vi "Read Asynchronous Measurement (Resistance).vi"(6 "Wait Time (10 S)":i32=10, 8 "error in (no error)":errorcluster, 9 "Resistance Buffer (smua.nvbuffer1)":string="smua.nvbuffer1", 10 "Source Measure Unit Channel (0: Channel A)":i32(ring) items=["Channel A", "Channel B"], 11 "VISA resource name":refnum<visa-resource-name>) -> (0 "error out":errorcluster, 2 "Resistance Buffer Data (Ohm)":dbl[](array[numeric]), 3 "VISA resource name out":refnum<visa-resource-name>)   [LabVIEW 2019, in "Keithley 2600 Series.lvlib"]
doc: "Returns the asynchronous resistance measurements."
uses:
  Keithley 2600 Series.lvlib
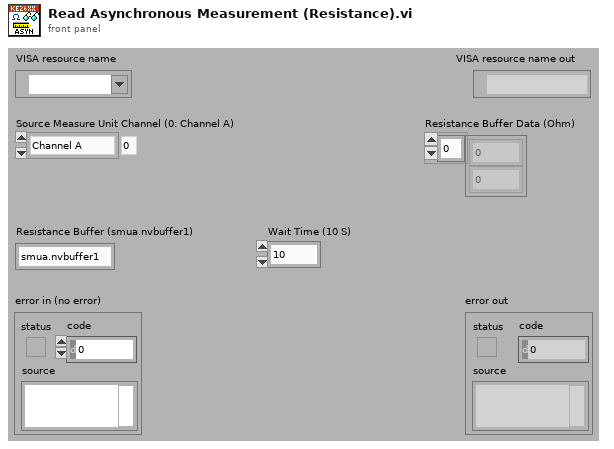
[diagram p1: front panel]
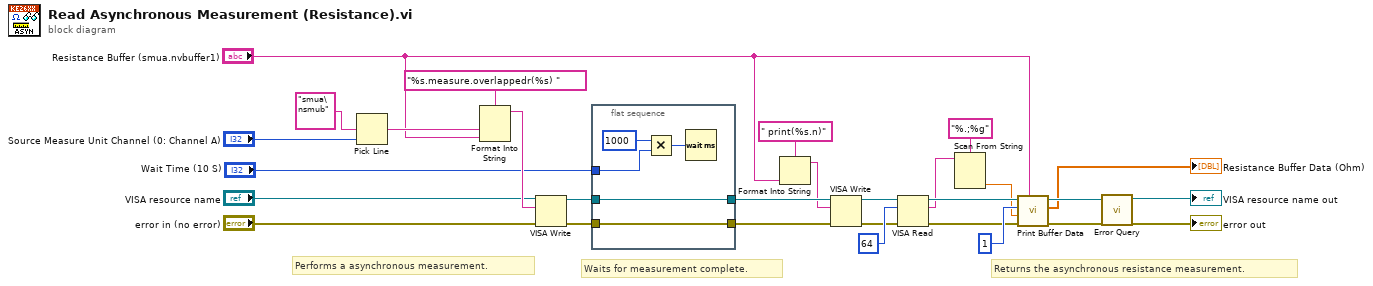
[diagram p0: block diagram]
diagram:
  # "Performs a asynchronous measurement."
  # "Waits for measurement complete."
  # "Returns the asynchronous resistance measurement."
  n1 = Pick Line(multi-line string="smua\nsmub", line index="Source Measure Unit Channel (0: Channel A)") -> (output string=w20:string)  [unwired: 1 in]
  n2 = Format Into String(format string="%s.measure.overlappedr(%s) ", w20, "Resistance Buffer (smua.nvbuffer1)") -> (resulting string=w26:string)  [unwired: 2 in, 1 out]
  n3 = VISA Write(VISA resource name="VISA resource name", write buffer=w26, error in (no error)="error in (no error)") -> (VISA resource name out=w10:refnum<visa-resource-name>, error out=w9:errorcluster)  [unwired: 1 out]
  n4 = flat-sequence {
    tunnel: w10 -> [w34]
    tunnel: w9 -> [w33]
    tunnel: [w34] -> w8
    tunnel: [w33] -> w7
    tunnel: "Wait Time (10 S)" -> [w32]
    frame #0 {
      n5 = Multiply(x=u32 1000, y=w32) -> (x*y=w30:u32)
      n6 = Wait (ms)(milliseconds to wait=w30) -> ()  [unwired: 1 out]
    }
  }
  n7 = Format Into String(format string=" print(%s.n)", "Resistance Buffer (smua.nvbuffer1)") -> (resulting string=w2:string)  [unwired: 2 in, 1 out]
  n8 = VISA Write(VISA resource name=w8, write buffer=w2, error in (no error)=w7) -> (VISA resource name out=w6:refnum<visa-resource-name>, error out=w5:errorcluster)  [unwired: 1 out]
  n9 = VISA Read(VISA resource name=w6, byte count=u32 64, error in (no error)=w5) -> (VISA resource name out=w23:refnum<visa-resource-name>, read buffer=w19:string, error out=w22:errorcluster)  [unwired: 1 out]
  n10 = Scan From String(format string="%.;%g", input string=w19) -> (output 1=w18:dbl)  [unwired: 3 in, 3 out]
  n11 = call "Print Buffer Data.vi"("Reading Buffer (smua.nvbuffer1)"="Resistance Buffer (smua.nvbuffer1)", "error in (no error)"=w22, "End Index (1)"=w18, "Start Index (1)"=1 ("Start Index (0)"), "VISA resource name"=w23) -> ("error out"=w12:errorcluster, "Buffer Data"=→"Resistance Buffer Data (Ohm)":dbl[], "VISA resource name out"=w13:refnum<visa-resource-name>)  [unwired: 4 in]
  n12 = call "Error Query.vi"("error in (no error)"=w12, "VISA resource name"=w13) -> ("error out"=→"error out":errorcluster, "VISA resource name out"=→"VISA resource name out":refnum<visa-resource-name>)  [unwired: 6 in, 2 out]
